vi "Check_Hysteresis.vi"(5 "Hall Sensor":bool, 6 "State In":enum16{"Check Threshold", "Bounce Time"}(ring), 7 "Bounce time (uSec)":u32 caption="Bounce Time (uSec)", 8 "Slope":enum16{"falling", "rising"}(ring)) -> (0 "State Out":enum16{"Check Threshold", "Bounce Time"}(ring), 1 "Event Ocurred?":bool)   [LabVIEW 2019]
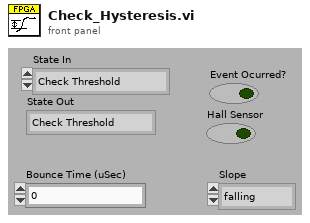
[diagram p1: front panel]
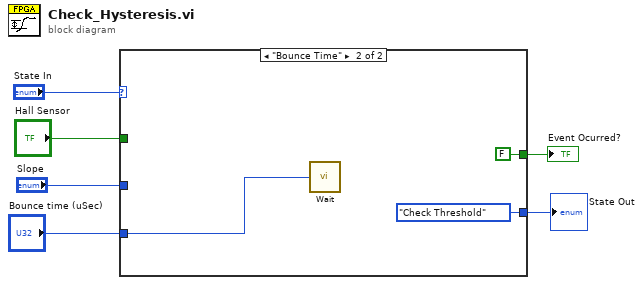
[diagram p0: block diagram]
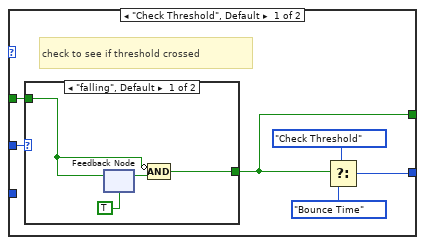
[diagram p2: hidden frame]
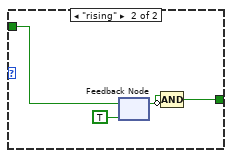
[diagram p3: hidden frame]
diagram:
  n1 = case shown="\"Bounce Time\"" "State In" {
    tunnel: [w10 enum16{"Check Threshold", "Bounce Time"}."Check Threshold" ("state")] -> w1
    tunnel: "Slope" -> [w12 _]
    tunnel: [w9 FALSE] -> w5
    tunnel: "Hall Sensor" -> [w8 _]
    tunnel: "Bounce time (uSec)" -> [_ w23]
    frame "Check Threshold", Default {
      # "check to see if threshold crossed"
      n2 = case shown="\"falling\", Default" w12 {
        tunnel: [w14 w18] -> w9
        tunnel: w8 -> [w13 w17]
        frame "falling", Default {
          n3 = feedback #1(TRUE) -> (w15:bool)
          n4 = feedback-in #1(w13) -> ()
          n5 = Compound Arithmetic op=AND(invert w13, w15) -> (w14:bool)
        }
        frame "rising" {
          n6 = feedback #2(TRUE) -> (w19:bool)
          n7 = feedback-in #2(w17) -> ()
          n8 = Compound Arithmetic op=AND(w17, invert w19) -> (w18:bool)
        }
      }
      n9 = Select(t=enum16{"Check Threshold", "Bounce Time"}."Check Threshold" ("state"), s=w9, f=enum16{"Check Threshold", "Bounce Time"}."Bounce Time" ("state")) -> (s? t:f=w10:enum16{"Check Threshold", "Bounce Time"})
    }
    frame "Bounce Time" {
      n10 = call "Wait"("Count(uSec)"=w23) -> ()  [unwired: 1 out]
    }
  }
  "Event Ocurred?" <- w5
  "State Out" <- w1
